vi "Write.vi"(8 "error in (no error)":errorcluster, 10 "Numeric":u8, 11 "Boolean in":refnum<class "conc_SharedVar_U8.lvclass">) -> (0 "error out":errorcluster, 3 "Boolean out":refnum<class "conc_SharedVar_U8.lvclass">)   [LabVIEW 2021, in "conc_SharedVar_U8.lvclass"]
doc: "LVabs_Shared Variable 1.0.0.2\nTim - TSA\nCopyright (c) 2024, TSA"
uses:
  conc_SharedVar_U8.lvclass
  conc_SharedVar_U8.lvclass/conc_SharedVar_U8.ctl
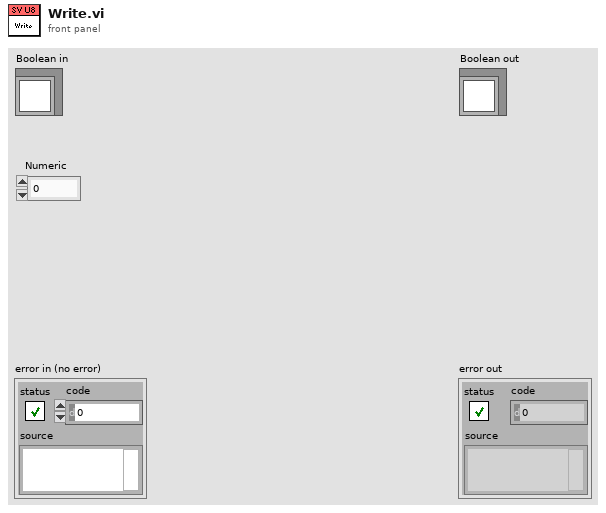
[diagram p1: front panel]
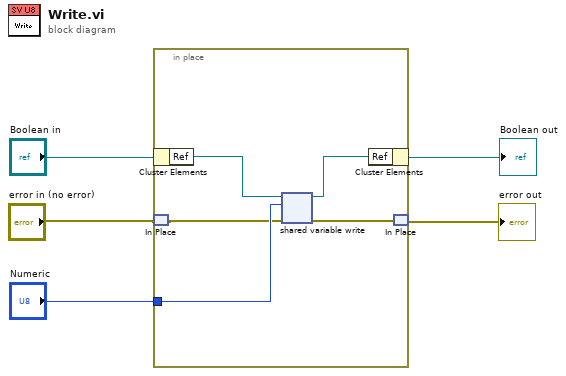
[diagram p0: block diagram]
diagram:
  n1 = in-place {
    in-place-border: "Numeric" -> [w8]
    n2 = in-place-cluster #1("Boolean in") -> ("Ref"=w10:refnum<k21>)
    n3 = in-place-match #2("error in (no error)") -> (w7:errorcluster)
    n4 = shared-variable-write(w10, w7, w8) -> (w9:refnum<k21>, w6:errorcluster)
    n5 = in-place-cluster #1("Ref"=w9) -> (→"Boolean out":refnum<class "conc_SharedVar_U8.lvclass">)
    n6 = in-place-match #2(w6) -> (→"error out":errorcluster)
  }
